vi "LV8 MIDI Throughput.vi"() -> ()   [LabVIEW 2014]
doc: "This VI inputs a \"MIDIshortmsg\" from the Windows OS, displays that message as a 32-bit integer and routes that message back to the Windows OS so that it may be played by the appropriate MIDI tone generator in the \"Sound and Audio Devices\" that are known to be available to the OS.\n\nSince the Windows OS uses \"callbacks\" to receive incoming MIDI data, a custom DLL (MIDIDLL.dll) has been included to receive this data and make it available to the LabVIEW VI. The LabVIEW program uses a custom \"Dynamic User Event\" and an \"Event Structure\" to retrieve the \"value\" of this MIDI data and pass it back to the OS for MIDI Output.\n\nThis program does not deal with MIDI \"System Exclusive\" messages and its operation if a SYSEX message is transmitted by the MIDI Input Device is currently unknown.\n\nThe four VI's in the MIDI Output data flow were taken from the \"midi-out example\" program that is available on the NI website.\n\nThe \"Tips and Descriptions\" for each control and indicator contain information specific to the use of items in this program."
uses:
  MIDI Voices.ctl
panel:
  in  "stop":bool
  out "output param":i32
  in  "MIDI Input Device":i32
  out "MIDI Short Message":i32 format="%08x"
  in  "MIDI Output Device":u32 max=10 step=1
  in  "patch?":T1
  out "Patch select error code":i32
  in  "channel":i32
  out "Close error code":i32
  out "Open error code":i32
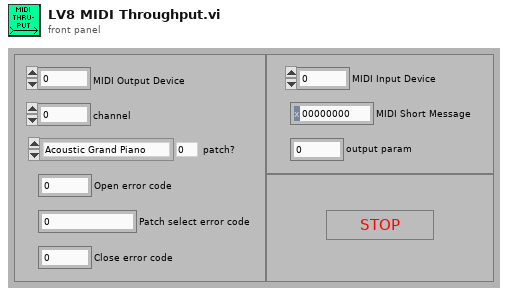
[diagram p1: front panel]
types:
  T1 = typedef "MIDI Voices.ctl" = enum32{"Acoustic Grand Piano", "Bright Acoustic Piano", "Electric Grand Piano", "Honky Tonk Piano", "Electric Piano 1", "Electric Piano 2", "Harpsichord", "Clavinet", "Celesta", "Glockenspiel", "Music Box", "Vibraphone", "Marimba", "Xylophone", "Tubular Bells", "Dulcimer", "Drawbar Organ", "Percussive Organ", "Rock Organ", "Church Organ", "Reed Organ", "Accordian", "Harmonica", "Tango Accordian", "Nylon Acoustic Guitar", "Steel Acoustic Guitar", "Jazz Electric Guitar", "Clean Electric Guitar", "Muted Electric Guitar", "Overdrive Guitar", "Distorted Guitar", "Harmonics Guitar", "Acoustic Bass", "Fingered Bass", "Electric Picked Bass", "Fretless Bass", "Slap Bass 1", "Slap Bass 2", "Synth Bass 1", "Synth Bass 2", "Violin", "Viola", "Cello", "Contrabass", "Tremelo Strings", "Pizzicato Strings", "Orchestral Harp", "Timpani", "String Ensemble 1", "String Ensemble 2", "Synth Strings 1", "Synth Strings 2", "Choir Aahs", "Voice Oohs", "Synth Choir", "Orchestral Hit", "Trumpet", "Trombone", "Tuba", "Muted Trumpet", "French Horn", "Synth Brass 1", "Synth Brass 2", "Synth Brass 3", "Soprano Sax", "Alto Sax", "Tenor Sax", "Baritone Sax", "Oboe", "English Horn", "Bassoon", "Clarinet", "Piccolo", "Flute", "Recorder", "Pan Flute", "Bottle Blow", "Shakuhachi", "Whistle", "Ocarina", "Synth Square Wave", "Synth Sawtooth Wave 1", "Synth Calliope", "Synth Chiff", "Synth Charanag", "Synth Voice", "Synth Sawtooth Wave 2", "Synth Brass & Lead", "New Age Synth Pad", "Warm Synth Pad", "Polysynth Synth Pad", "Choir Synth Pad", "Bowed Synth Pad", "Metal Synth Pad", "Halo Synth Pad", "Sweep Synth Pad", "SFX Rain", "SFX Soundtrack", "SFX Crystal", "SFX Atmosphere", "SFX Brightness", "SFX Goblins", "SFX Echoes", "SFX Sci-Fi", "Sitar", "Banjo", "Shamisen", "Koto", "Kalimba", "Bag Pipe", "Fiddle", "Shanai", "Tinkle Bell", "Agogo", "Steel Drums", "Woodblock", "Taiko Drum", "Melodic Tom", "Synth Drum", "Reverse Cymbal", "Guitar Fret Noise", "Breath Noise", "Seashore", "Bird Tweet", "Telephone Ring", "Helicopter", "Applause", "Gun Shot"}
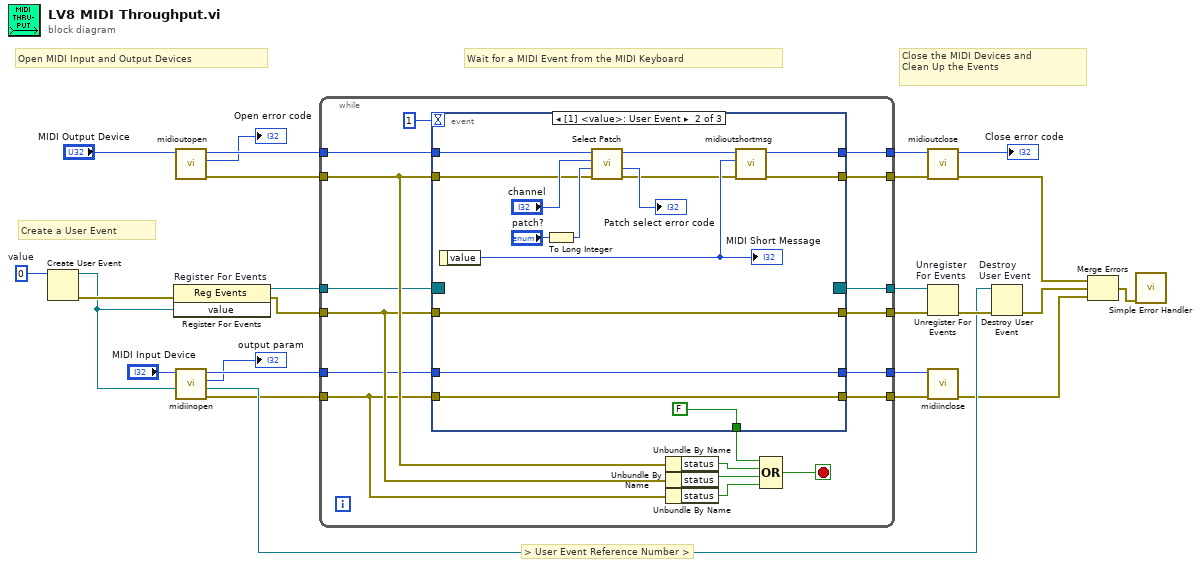
[diagram p0: block diagram]
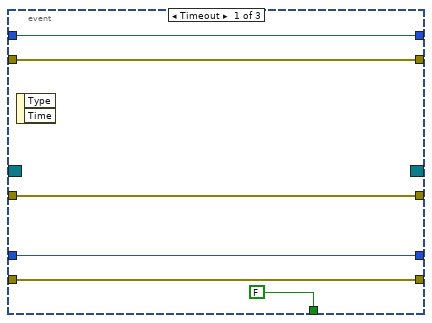
[diagram p2: hidden frame]
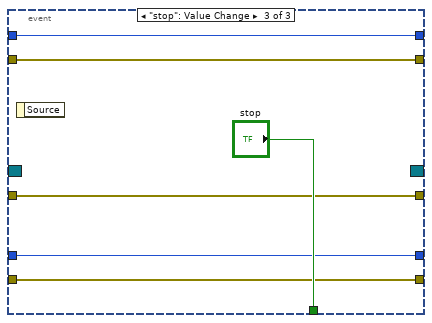
[diagram p3: hidden frame]
diagram:
  w26 = 0  # value
  # "Create a User Event"
  # "Close the MIDI Devices and\nClean Up the Events"
  # "Wait for a MIDI Event from the MIDI Keyboard"
  # "Open MIDI Input and Output Devices"
  # "> User Event Reference Number >"
  n1 = Create User Event(user event datatype=w26) -> (user event=w7:refnum<user-event>, error out=w22:errorcluster)  [unwired: 1 in]
  n2 = register-events "Register For Events"(error in=w22, w7) -> (reference out=w25:refnum<event-registration>, error out=w16:errorcluster)  [unwired: 1 in]
  n3 = call "midioutopen.vi"("uDeviceID"="MIDI Output Device") -> ("error out"=w15:errorcluster, "Win32 Error Code"=→"Open error code":i32, "hmidiout handle"=w18:i32)  [unwired: 4 in]
  n4 = call "midiinopen.vi"("value"=w7, "MIDI Input Device"="MIDI Input Device") -> ("error out"=w4:errorcluster, "value out"=w6:refnum<user-event>, "output param"=→"output param":i32, "hmidiin"=w8:i32)  [unwired: 2 in]
  n5 = while {
    tunnel: w25 -> [w28]
    tunnel: w16 -> [w36]
    tunnel: [w44] -> w21
    tunnel: [w43] -> w24
    tunnel: w8 -> [w27]
    tunnel: [w42] -> w19
    tunnel: w18 -> [w41]
    tunnel: [w40] -> w3
    tunnel: w15 -> [w37]
    tunnel: [w39] -> w12
    tunnel: w4 -> [w35]
    tunnel: [w38] -> w2
    stop <- w30 stop-if-true
    n6 = event shown="[1] <value>: User Event" {
      selector: w28 -> [_ _ _]
      dyn-events: [_ _ _] -> w43
      timeout: 1 -> [_ _ _]
      tunnel: [FALSE ("stop") FALSE ("stop") "stop"] -> w31
      tunnel: w36 -> [w48 w64 w69]
      tunnel: [w48 w64 w69] -> w44
      tunnel: w27 -> [w47 w59 w68]
      tunnel: w41 -> [w49 w61 w70]
      tunnel: [w49 w55 w70] -> w42
      tunnel: [w47 w59 w68] -> w40
      tunnel: w37 -> [w46 w57 w67]
      tunnel: [w46 w52 w67] -> w39
      tunnel: w35 -> [w45 w51 w66]
      tunnel: [w45 w51 w66] -> w38
      event Timeout {
        n7 = event-data() -> ()  [unwired: 1 in, 2 out]
      }
      event User Event {
        n8 = event-data() -> ("value"=w54:i32)  [unwired: 1 in]
        "MIDI Short Message" <- w54
        n9 = To Long Integer(number="patch?") -> (32bit integer=w60:i32)
        n10 = call "Select Patch.vi"("error in (no error)"=w57, "patch?"=w60, "channel"="channel", "MIDI out handle"=w61) -> ("error out"=w53:errorcluster, "Win32 error code"=→"Patch select error code":i32, "duplicate MIDI handle"=w56:i32)  [unwired: 1 in]
        n11 = call "midioutshortmsg.vi"("error in (no error)"=w53, "data"=w54, "MIDI output handle"=w56) -> ("error out"=w52:errorcluster, "duplicate MIDI output handle"=w55:i32)  [unwired: 2 in, 1 out]
      }
      event "stop": Value Change {
        n12 = event-data() -> ()  [unwired: 1 in, 1 out]
      }
    }
    n13 = Unbundle By Name(w37) -> ("status"=w34:bool)
    n14 = Unbundle By Name(w36) -> ("status"=w33:bool)
    n15 = Unbundle By Name(w35) -> ("status"=w32:bool)
    n16 = Compound Arithmetic op=OR(w31, w34, w33, w32) -> (w30:bool)
  }
  n17 = call "midioutclose.vi"("error in (no error)"=w12, "MIDI output handle"=w19) -> ("error out"=w10:errorcluster, "Win32 error code"=→"Close error code":i32)  [unwired: 4 in]
  n18 = Unregister For Events "Unregister\nFor Events"(event registration refnum=w24, error in=w21) -> (error out=w23:errorcluster)
  n19 = call "midiinclose.vi"("error in (no error)"=w2, "hmidiin"=w3) -> ("error out"=w1:errorcluster)  [unwired: 4 in, 1 out]
  n20 = Destroy User Event "Destroy\nUser Event"(user event=w6, error in=w23) -> (error out=w14:errorcluster)
  n21 = Merge Errors(w10, w14, w1) -> (w13:errorcluster)
  n22 = call <vilib>:"Simple Error Handler.vi"("error in (no error)"=w13) -> ()  [unwired: 4 in, 5 out]
